vi "DestroyMessageQueues.vi"(8 "error in":errorcluster, 11 "message ref in":refnum<class "CLM_PriorityLocalMessage.lvclass">) -> (0 "error out":errorcluster, 2 "remaining elements":T1[](array[typedef]))   [LabVIEW 2013, in "CLM_PriorityLocalMessage.lvclass"]
uses:
  CLM_PriorityLocalMessage.lvclass
  LocalMessage/Message.ctl
  CLM_PriorityLocalMessage.lvclass/CLM_PriorityLocalMessage.ctl
  FG_NamedQueuesAction.ctl
  LocalMessage_Queue/CLM_LocalMessage_Queue.lvclass/CLM_LocalMessage_Queue.ctl
  LocalMessage_Queue/CLM_LocalMessage_Queue.lvclass
  LocalMessage/CLM_LocalMessage.lvclass
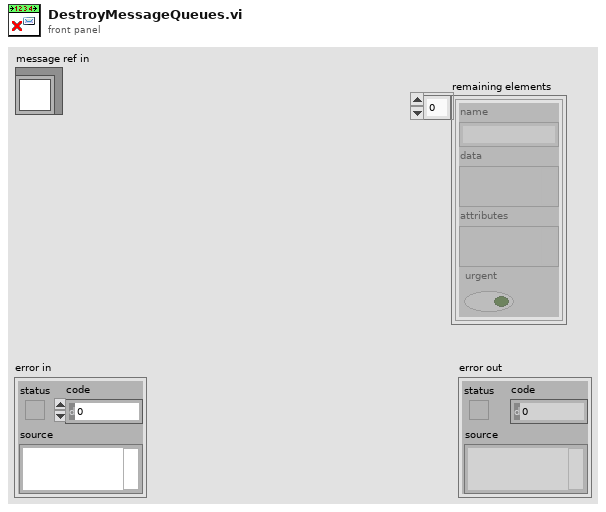
[diagram p1: front panel]
types:
  T1 = typedef "CLM_LocalMessage.lvclass/Message.ctl" = cluster{"name":string, "data":variant, "attributes":variant, "urgent":bool}
  T2 = typedef "CLM_PriorityLocalMessage.lvclass/FG_NamedQueuesAction.ctl" = enum16{"Get", "Add", "Remove", "RemoveAll"}
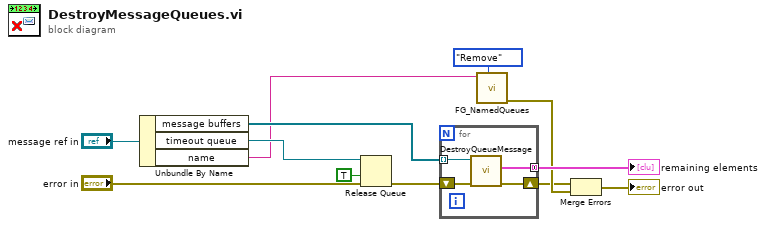
[diagram p0: block diagram]
diagram:
  n1 = Unbundle By Name("message ref in") -> ("message buffers"=w11:refnum<class "CLM_LocalMessage_Queue.lvclass">[], "timeout queue"=w9:refnum<queue>, "name"=w5:string)
  n2 = Release Queue(queue=w9, force destroy? (F)=TRUE, error in (no error)="error in") -> (error out=w8:errorcluster)  [unwired: 2 out]
  n3 = for {
    tunnel: w11 -> [w16] mode=indexing
    tunnel: [w15] -> w10 mode=concatenating
    shift-right: [w14] -> w2
    shift-left: w8 -> [w13]
    n4 = call "DestroyQueueMessage.vi"("error in"=w13, "message ref in"=w16) -> ("error out"=w14:errorcluster, "remaining elements"=w15:T1[])  [unwired: 8 in]
  }
  "remaining elements" <- w10
  n5 = call "FG_NamedQueues.vi"("action"=FG_NamedQueuesAction."Remove", "name"=w5) -> ("error out"=w3:errorcluster)  [unwired: 7 in, 2 out]
  n6 = Merge Errors(w2, w3) -> (→"error out":errorcluster)
